vi "Invert eqaution.vi"(1 "Distance":dbl, 2 "Height":dbl) -> (0 "Calculated Zavit":dbl)   [LabVIEW 2012]
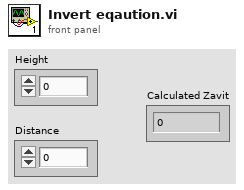
[diagram p1: front panel]
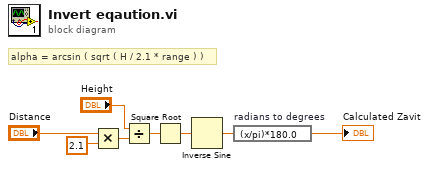
[diagram p0: block diagram]
diagram:
  # "alpha = arcsin ( sqrt ( H / 2.1 * range ) )"
  n1 = Multiply(x="Distance", y=2.1 ("value")) -> (x*y=w4:dbl)
  n2 = Divide(x="Height", y=w4) -> (x/y=w1:dbl)
  n3 = Square Root(x=w1) -> (sqrt(x)=w6:dbl)
  n4 = Inverse Sine(1:w6) -> (0:w8:dbl)
  n5 = expression code="(x/pi)*180.0" "radians to degrees"(w8) -> (→"Calculated Zavit":dbl)
